vi "Get Enum Size.vi"(1 "Enum":T1=enum."Recording Duration") -> (0 "Size":i32)   [LabVIEW 2020]
uses:
  Control/Execute - Index of Elapse time.ctl
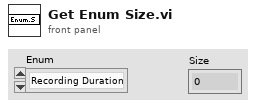
[diagram p1: front panel]
types:
  T1 = typedef "Execute - Index of Elapse time.ctl" = enum16{"Elapse Gap Data", "Holding Time", "Recording Duration", "View Change", "Pressure stabilize timer", "Press. Drop Rate", "Init Holding Buffer"}
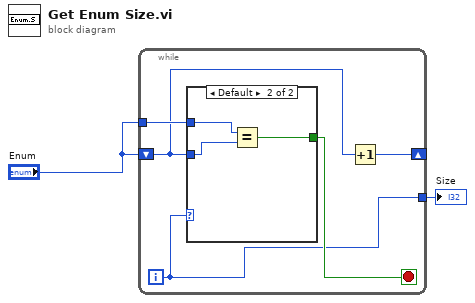
[diagram p0: block diagram]
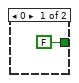
[diagram p2: hidden frame]
diagram:
  n1 = while {
    shift-right: [w3] -> _
    shift-left: "Enum" -> [w4]
    tunnel: "Enum" -> [w7]
    tunnel: [w5] -> w1
    i -> [w5]
    stop <- w6 stop-if-true
    n2 = case shown="Default" w5 {
      tunnel: w4 -> [_ w10]
      tunnel: w7 -> [_ w11]
      tunnel: [FALSE w9] -> w6
      frame 0 {
      }
      frame Default {
        n3 = Equal?(x=w11, y=w10) -> (x = y?=w9:bool)
      }
    }
    n4 = Increment(x=w4) -> (x+1=w3:T1)
  }
  "Size" <- w1
